vi "SysCfgGetPackagesResponse_Parse.vi"(10 "Message":T2) -> (2 "output cluster":T1)   [LabVIEW 2016]
uses:
  <vilib>/addons/InsightCM/MessageBus/Base/controls/KeyValuePair.ctl
  <vilib>/addons/InsightCM/MessageBus/Base/controls/MessageHeader.ctl
  <vilib>/addons/InsightCM/MessageBus/Base/controls/Message.ctl
panel:
  out "error out":errorcluster
  in  "error in (no error)":errorcluster
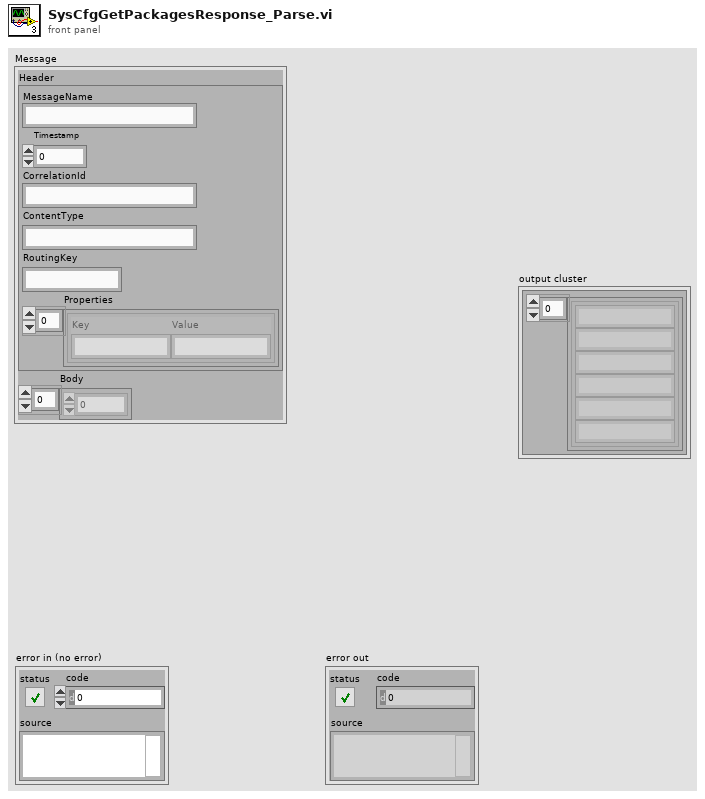
[diagram p1: front panel]
types:
  T1 = cluster{cluster{cluster{string, string, string, string, string, string}[]}}
  T2 = typedef "Message.ctl" = cluster{"Header":T3, "Body":u8[]}
  T3 = typedef "MessageHeader.ctl" = cluster{"MessageName":string, "Timestamp":i64, "CorrelationId":string, "ContentType":string, "RoutingKey":string, "Properties":T4[]}
  T4 = typedef "KeyValuePair.ctl" = cluster{"Key":string, "Value":string}
  T5 = cluster{cluster{string, string, string, string, string, string}[]}
  T6 = cluster{string, string, string, string, string, string}
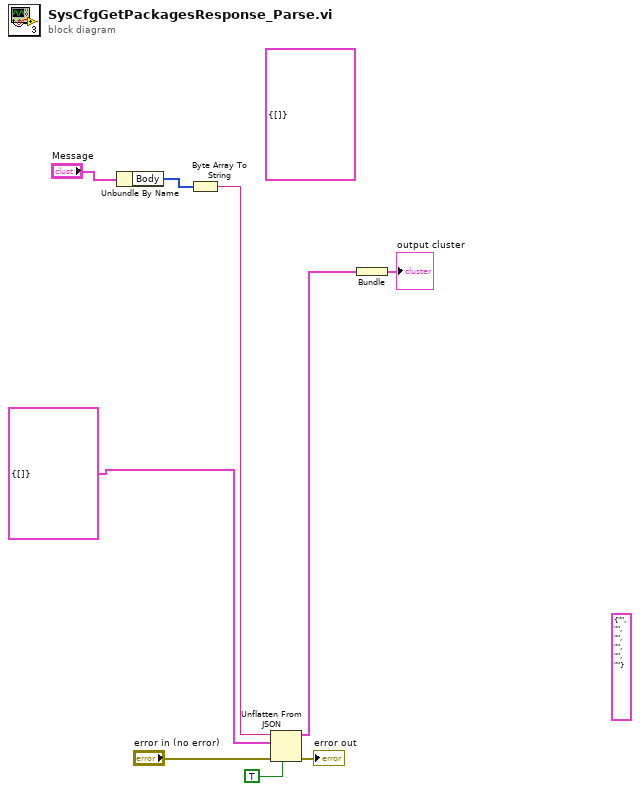
[diagram p0: block diagram]
diagram:
  (unwired) T6 {"", "", "", "", "", ""}
  (unwired) T5 {[]}
  n1 = Unbundle By Name("Message") -> ("Body"=w4:u8[])
  n2 = Byte Array To String(unsigned byte array=w4) -> (string=w6:string)
  n3 = Unflatten From JSON(JSON string=w6, type and defaults=T5 {[]}, default null elements? (F)=TRUE, error in (no error)="error in (no error)") -> (value=w2:T5, error out=→"error out":errorcluster)  [unwired: 3 in]
  n4 = Bundle(w2) -> (→"output cluster":T1)  [unwired: 1 in]
